vi "json_template_openweather.vi"() -> ()   [LabVIEW 2020]
panel:
  in  "?":T1
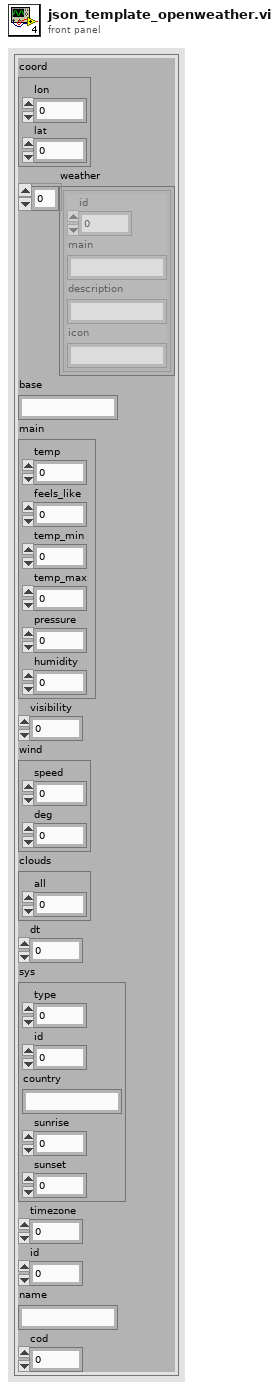
[diagram p1: front panel]
types:
  T1 = cluster{"coord":cluster{"lon":dbl, "lat":dbl}, "weather":cluster{"id":i32, "main":string, "description":string, "icon":string}[], "base":string, "main":cluster{"temp":i32, "feels_like":i32, "temp_min":i32, "temp_max":i32, "pressure":i32, "humidity":i32}, "visibility":i32, "wind":cluster{"speed":i32, "deg":i32}, "clouds":cluster{"all":i32}, "dt":i32, "sys":cluster{"type":i32, "id":i32, "country":string, "sunrise":i32, "sunset":i32}, "timezone":i32, "id":i32, "name":string, "cod":i32}
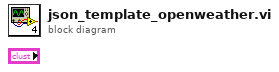
[diagram p0: block diagram]
diagram:
